vi "fftw__memcpy_from_real_poly.vi"   [LabVIEW 2020, in "FFTWDLL.lvlib"]
doc: "Copy LV real array to FFTW aligned array."
uses:
  FFTWDLL.lvlib
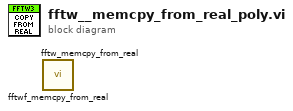
[diagram p0: block diagram]
diagram:
  n1 = call "fftwf_memcpy_from_real.vi"() -> ()  [unwired: 10 in, 2 out]
  n2 = call "fftw_memcpy_from_real.vi"() -> ()  [unwired: 10 in, 2 out]
